vi "GetTaskStatus.vi"(8 "error in (no error)":errorcluster, 10 "task":i32, 11 "controller in":refnum<k24>) -> (0 "error out":errorcluster, 2 "task status":T1, 3 "controller out":refnum<k24>)   [LabVIEW 2010]
uses:
  c:/aerotech/controller/5.xx.xxx/A3200/pc/labview/2010/bin/Aerotech.A3200.dll
  bin/Aerotech.A3200.dll
  TaskStatus.ctl
  c:/aerotech/controller/5.xx.xxx/A3200/pc/labview/2010/bin/Aerotech.A3200.LabVIEW.dll
  bin/Aerotech.A3200.LabVIEW.dll
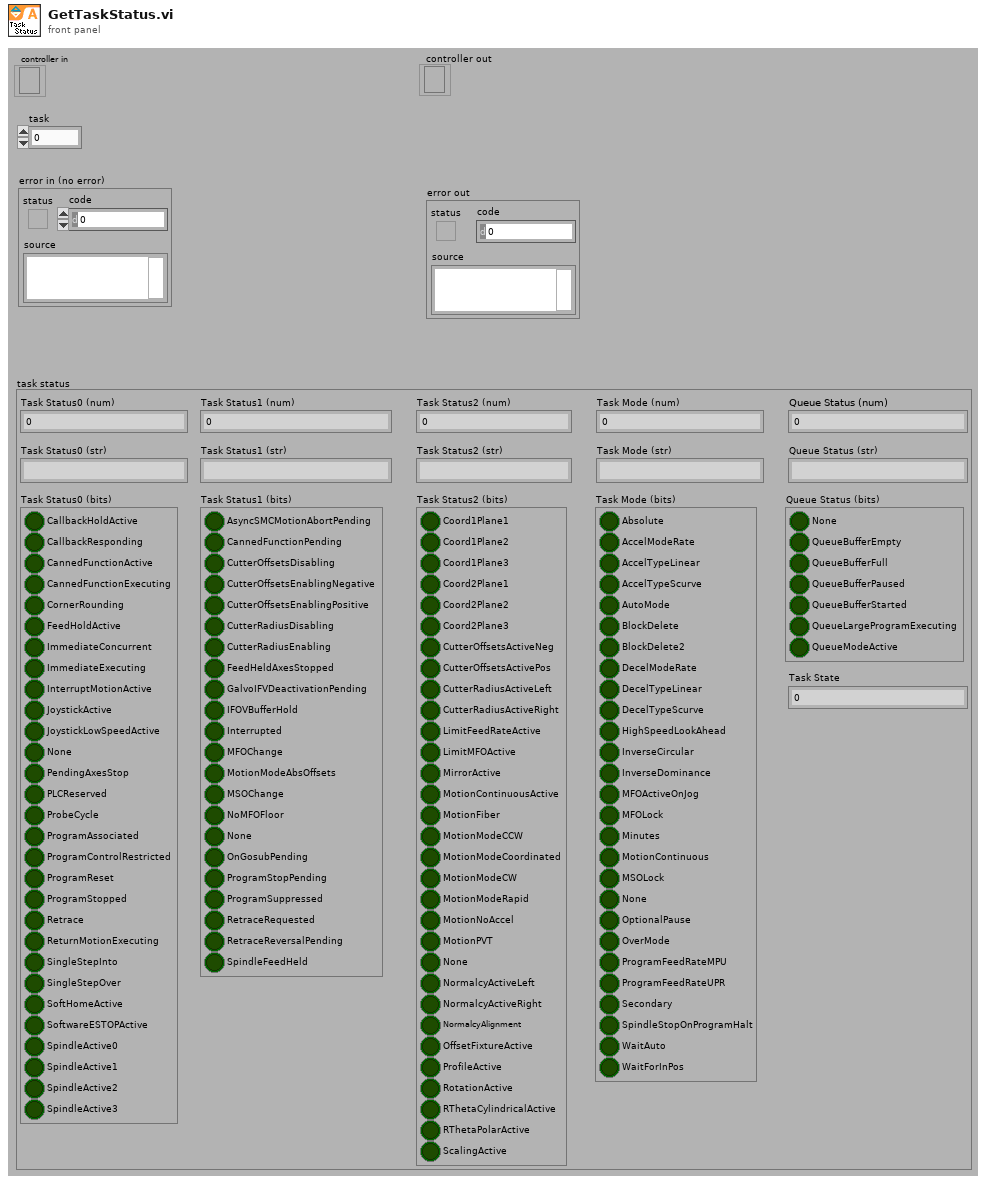
[diagram p1: front panel]
types:
  T1 = typedef "TaskStatus.ctl" = cluster{"Task Status0 (num)":i32, "Task Status0 (bits)":cluster{"CallbackHoldActive":bool, "CallbackResponding":bool, "CannedFunctionActive":bool, "CannedFunctionExecuting":bool, "CornerRounding":bool, "FeedHoldActive":bool, "ImmediateConcurrent":bool, "ImmediateExecuting":bool, "InterruptMotionActive":bool, "JoystickActive":bool, "JoystickLowSpeedActive":bool, "None":bool, "PendingAxesStop":bool, "PLCReserved":bool, "ProbeCycle":bool, "ProgramAssociated":bool, "ProgramControlRestricted":bool, "ProgramReset":bool, "ProgramStopped":bool, "Retrace":bool, "ReturnMotionExecuting":bool, "SingleStepInto":bool, "SingleStepOver":bool, "SoftHomeActive":bool, "SoftwareESTOPActive":bool, "SpindleActive0":bool, "SpindleActive1":bool, "SpindleActive2":bool, "SpindleActive3":bool}, "Task Status0 (str)":string, "Task Status1 (num)":i32, "Task Status1 (bits)":cluster{"AsyncSMCMotionAbortPending":bool, "CannedFunctionPending":bool, "CutterOffsetsDisabling":bool, "CutterOffsetsEnablingNegative":bool, "CutterOffsetsEnablingPositive":bool, "CutterRadiusDisabling":bool, "CutterRadiusEnabling":bool, "FeedHeldAxesStopped":bool, "GalvoIFVDeactivationPending":bool, "IFOVBufferHold":bool, "Interrupted":bool, "MFOChange":bool, "MotionModeAbsOffsets":bool, "MSOChange":bool, "NoMFOFloor":bool, "None":bool, "OnGosubPending":bool, "ProgramStopPending":bool, "ProgramSuppressed":bool, "RetraceRequested":bool, "RetraceReversalPending":bool, "SpindleFeedHeld":bool}, "Task Status1 (str)":string, "Task Status2 (num)":i32, "Task Status2 (bits)":cluster{"Coord1Plane1":bool, "Coord1Plane2":bool, "Coord1Plane3":bool, "Coord2Plane1":bool, "Coord2Plane2":bool, "Coord2Plane3":bool, "CutterOffsetsActiveNeg":bool, "CutterOffsetsActivePos":bool, "CutterRadiusActiveLeft":bool, "CutterRadiusActiveRight":bool, "LimitFeedRateActive":bool, "LimitMFOActive":bool, "MirrorActive":bool, "MotionContinuousActive":bool, "MotionFiber":bool, "MotionModeCCW":bool, "MotionModeCoordinated":bool, "MotionModeCW":bool, "MotionModeRapid":bool, "MotionNoAccel":bool, "MotionPVT":bool, "None":bool, "NormalcyActiveLeft":bool, "NormalcyActiveRight":bool, "NormalcyAlignment":bool, "OffsetFixtureActive":bool, "ProfileActive":bool, "RotationActive":bool, "RThetaCylindricalActive":bool, "RThetaPolarActive":bool, "ScalingActive":bool}, "Task Status2 (str)":string, "Task Mode (num)":i32, "Task Mode (bits)":cluster{"Absolute":bool, "AccelModeRate":bool, "AccelTypeLinear":bool, "AccelTypeScurve":bool, "AutoMode":bool, "BlockDelete":bool, "BlockDelete2":bool, "DecelModeRate":bool, "DecelTypeLinear":bool, "DecelTypeScurve":bool, "HighSpeedLookAhead":bool, "InverseCircular":bool, "InverseDominance":bool, "MFOActiveOnJog":bool, "MFOLock":bool, "Minutes":bool, "MotionContinuous":bool, "MSOLock":bool, "None":bool, "OptionalPause":bool, "OverMode":bool, "ProgramFeedRateMPU":bool, "ProgramFeedRateUPR":bool, "Secondary":bool, "SpindleStopOnProgramHalt":bool, "WaitAuto":bool, "WaitForInPos":bool}, "Task Mode (str)":string, "Queue Status (num)":i32, "Queue Status (bits)":cluster{"None":bool, "QueueBufferEmpty":bool, "QueueBufferFull":bool, "QueueBufferPaused":bool, "QueueBufferStarted":bool, "QueueLargeProgramExecuting":bool, "QueueModeActive":bool}, "Queue Status (str)":string, "Task State":i32}
  T2 = cluster{"taskStatus0Bits[0]":bool, "taskStatus0Bits[1]":bool, "taskStatus0Bits[2]":bool, "taskStatus0Bits[3]":bool, "taskStatus0Bits[4]":bool, "taskStatus0Bits[5]":bool, "taskStatus0Bits[6]":bool, "taskStatus0Bits[7]":bool, "taskStatus0Bits[8]":bool, "taskStatus0Bits[9]":bool, "taskStatus0Bits[10]":bool, "taskStatus0Bits[11]":bool, "taskStatus0Bits[12]":bool, "taskStatus0Bits[13]":bool, "taskStatus0Bits[14]":bool, "taskStatus0Bits[15]":bool, "taskStatus0Bits[16]":bool, "taskStatus0Bits[17]":bool, "taskStatus0Bits[18]":bool, "taskStatus0Bits[19]":bool, "taskStatus0Bits[20]":bool, "taskStatus0Bits[21]":bool, "taskStatus0Bits[22]":bool, "taskStatus0Bits[23]":bool, "taskStatus0Bits[24]":bool, "taskStatus0Bits[25]":bool, "taskStatus0Bits[26]":bool, "taskStatus0Bits[27]":bool, "taskStatus0Bits[28]":bool}
  T3 = cluster{"taskStatus1Bits[0]":bool, "taskStatus1Bits[1]":bool, "taskStatus1Bits[2]":bool, "taskStatus1Bits[3]":bool, "taskStatus1Bits[4]":bool, "taskStatus1Bits[5]":bool, "taskStatus1Bits[6]":bool, "taskStatus1Bits[7]":bool, "taskStatus1Bits[8]":bool, "taskStatus1Bits[9]":bool, "taskStatus1Bits[10]":bool, "taskStatus1Bits[11]":bool, "taskStatus1Bits[12]":bool, "taskStatus1Bits[13]":bool, "taskStatus1Bits[14]":bool, "taskStatus1Bits[15]":bool, "taskStatus1Bits[16]":bool, "taskStatus1Bits[17]":bool, "taskStatus1Bits[18]":bool, "taskStatus1Bits[19]":bool, "taskStatus1Bits[20]":bool, "taskStatus1Bits[21]":bool}
  T4 = cluster{"taskStatus2Bits[0]":bool, "taskStatus2Bits[1]":bool, "taskStatus2Bits[2]":bool, "taskStatus2Bits[3]":bool, "taskStatus2Bits[4]":bool, "taskStatus2Bits[5]":bool, "taskStatus2Bits[6]":bool, "taskStatus2Bits[7]":bool, "taskStatus2Bits[8]":bool, "taskStatus2Bits[9]":bool, "taskStatus2Bits[10]":bool, "taskStatus2Bits[11]":bool, "taskStatus2Bits[12]":bool, "taskStatus2Bits[13]":bool, "taskStatus2Bits[14]":bool, "taskStatus2Bits[15]":bool, "taskStatus2Bits[16]":bool, "taskStatus2Bits[17]":bool, "taskStatus2Bits[18]":bool, "taskStatus2Bits[19]":bool, "taskStatus2Bits[20]":bool, "taskStatus2Bits[21]":bool, "taskStatus2Bits[22]":bool, "taskStatus2Bits[23]":bool, "taskStatus2Bits[24]":bool, "taskStatus2Bits[25]":bool, "taskStatus2Bits[26]":bool, "taskStatus2Bits[27]":bool, "taskStatus2Bits[28]":bool, "taskStatus2Bits[29]":bool, "taskStatus2Bits[30]":bool}
  T5 = cluster{"taskModeBits[0]":bool, "taskModeBits[1]":bool, "taskModeBits[2]":bool, "taskModeBits[3]":bool, "taskModeBits[4]":bool, "taskModeBits[5]":bool, "taskModeBits[6]":bool, "taskModeBits[7]":bool, "taskModeBits[8]":bool, "taskModeBits[9]":bool, "taskModeBits[10]":bool, "taskModeBits[11]":bool, "taskModeBits[12]":bool, "taskModeBits[13]":bool, "taskModeBits[14]":bool, "taskModeBits[15]":bool, "taskModeBits[16]":bool, "taskModeBits[17]":bool, "taskModeBits[18]":bool, "taskModeBits[19]":bool, "taskModeBits[20]":bool, "taskModeBits[21]":bool, "taskModeBits[22]":bool, "taskModeBits[23]":bool, "taskModeBits[24]":bool, "taskModeBits[25]":bool, "taskModeBits[26]":bool}
  T6 = cluster{"queueStatusBits[0]":bool, "queueStatusBits[1]":bool, "queueStatusBits[2]":bool, "queueStatusBits[3]":bool, "queueStatusBits[4]":bool, "queueStatusBits[5]":bool, "queueStatusBits[6]":bool}
  T7 = cluster{"taskStatus0MaskValue":i32, "taskStatus0Bits":cluster{"taskStatus0Bits[0]":bool, "taskStatus0Bits[1]":bool, "taskStatus0Bits[2]":bool, "taskStatus0Bits[3]":bool, "taskStatus0Bits[4]":bool, "taskStatus0Bits[5]":bool, "taskStatus0Bits[6]":bool, "taskStatus0Bits[7]":bool, "taskStatus0Bits[8]":bool, "taskStatus0Bits[9]":bool, "taskStatus0Bits[10]":bool, "taskStatus0Bits[11]":bool, "taskStatus0Bits[12]":bool, "taskStatus0Bits[13]":bool, "taskStatus0Bits[14]":bool, "taskStatus0Bits[15]":bool, "taskStatus0Bits[16]":bool, "taskStatus0Bits[17]":bool, "taskStatus0Bits[18]":bool, "taskStatus0Bits[19]":bool, "taskStatus0Bits[20]":bool, "taskStatus0Bits[21]":bool, "taskStatus0Bits[22]":bool, "taskStatus0Bits[23]":bool, "taskStatus0Bits[24]":bool, "taskStatus0Bits[25]":bool, "taskStatus0Bits[26]":bool, "taskStatus0Bits[27]":bool, "taskStatus0Bits[28]":bool}, "taskStatus0String":string, "taskStatus1MaskValue":i32, "taskStatus1Bits":cluster{"taskStatus1Bits[0]":bool, "taskStatus1Bits[1]":bool, "taskStatus1Bits[2]":bool, "taskStatus1Bits[3]":bool, "taskStatus1Bits[4]":bool, "taskStatus1Bits[5]":bool, "taskStatus1Bits[6]":bool, "taskStatus1Bits[7]":bool, "taskStatus1Bits[8]":bool, "taskStatus1Bits[9]":bool, "taskStatus1Bits[10]":bool, "taskStatus1Bits[11]":bool, "taskStatus1Bits[12]":bool, "taskStatus1Bits[13]":bool, "taskStatus1Bits[14]":bool, "taskStatus1Bits[15]":bool, "taskStatus1Bits[16]":bool, "taskStatus1Bits[17]":bool, "taskStatus1Bits[18]":bool, "taskStatus1Bits[19]":bool, "taskStatus1Bits[20]":bool, "taskStatus1Bits[21]":bool}, "taskStatus1String":string, "taskStatus2MaskValue":i32, "taskStatus2Bits":cluster{"taskStatus2Bits[0]":bool, "taskStatus2Bits[1]":bool, "taskStatus2Bits[2]":bool, "taskStatus2Bits[3]":bool, "taskStatus2Bits[4]":bool, "taskStatus2Bits[5]":bool, "taskStatus2Bits[6]":bool, "taskStatus2Bits[7]":bool, "taskStatus2Bits[8]":bool, "taskStatus2Bits[9]":bool, "taskStatus2Bits[10]":bool, "taskStatus2Bits[11]":bool, "taskStatus2Bits[12]":bool, "taskStatus2Bits[13]":bool, "taskStatus2Bits[14]":bool, "taskStatus2Bits[15]":bool, "taskStatus2Bits[16]":bool, "taskStatus2Bits[17]":bool, "taskStatus2Bits[18]":bool, "taskStatus2Bits[19]":bool, "taskStatus2Bits[20]":bool, "taskStatus2Bits[21]":bool, "taskStatus2Bits[22]":bool, "taskStatus2Bits[23]":bool, "taskStatus2Bits[24]":bool, "taskStatus2Bits[25]":bool, "taskStatus2Bits[26]":bool, "taskStatus2Bits[27]":bool, "taskStatus2Bits[28]":bool, "taskStatus2Bits[29]":bool, "taskStatus2Bits[30]":bool}, "taskStatus2String":string, "taskModeMaskValue":i32, "taskModeBits":cluster{"taskModeBits[0]":bool, "taskModeBits[1]":bool, "taskModeBits[2]":bool, "taskModeBits[3]":bool, "taskModeBits[4]":bool, "taskModeBits[5]":bool, "taskModeBits[6]":bool, "taskModeBits[7]":bool, "taskModeBits[8]":bool, "taskModeBits[9]":bool, "taskModeBits[10]":bool, "taskModeBits[11]":bool, "taskModeBits[12]":bool, "taskModeBits[13]":bool, "taskModeBits[14]":bool, "taskModeBits[15]":bool, "taskModeBits[16]":bool, "taskModeBits[17]":bool, "taskModeBits[18]":bool, "taskModeBits[19]":bool, "taskModeBits[20]":bool, "taskModeBits[21]":bool, "taskModeBits[22]":bool, "taskModeBits[23]":bool, "taskModeBits[24]":bool, "taskModeBits[25]":bool, "taskModeBits[26]":bool}, "taskModeString":string, "queueStatusMaskValue":i32, "queueStatusBits":cluster{"queueStatusBits[0]":bool, "queueStatusBits[1]":bool, "queueStatusBits[2]":bool, "queueStatusBits[3]":bool, "queueStatusBits[4]":bool, "queueStatusBits[5]":bool, "queueStatusBits[6]":bool}, "queueStatusString":string, "taskState":i32}
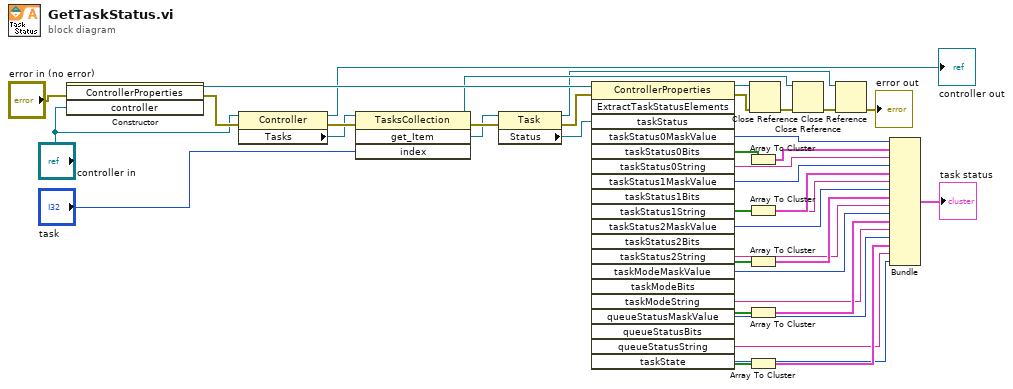
[diagram p0: block diagram]
diagram:
  n1 = constructor class="ControllerProperties"(error in="error in (no error)", "controller"="controller in") -> (reference out=w40:refnum<k24>, error out=w39:errorcluster)  [unwired: 2 in, 2 out]
  n2 = property class="Controller"(reference="controller in", error in=w39) -> (reference out=→"controller out":refnum<k24>, error out=w37:errorcluster, "Tasks"=w9:refnum<k24>)
  n3 = invoke class="TasksCollection" method="get_Item"(reference=w9, error in=w37, "index"="task") -> (reference out=w5:refnum<k24>, error out=w35:errorcluster, "get_Item"=w34:refnum<k24>)  [unwired: 1 in, 1 out]
  n4 = property class="Task"(reference=w34, error in=w35) -> (reference out=w4:refnum<k24>, error out=w32:errorcluster, "Status"=w33:refnum<k24>)
  n5 = invoke class="ControllerProperties" method="ExtractTaskStatusElements"(reference=w40, error in=w32, "taskStatus"=w33) -> (reference out=w7:refnum<k24>, error out=w6:errorcluster, "taskStatus0MaskValue"=w31:i32, "taskStatus0Bits"=w30:bool[], "taskStatus0String"=w24:string, "taskStatus1MaskValue"=w23:i32, "taskStatus1Bits"=w29:bool[], "taskStatus1String"=w21:string, "taskStatus2MaskValue"=w20:i32, "taskStatus2Bits"=w28:bool[], "taskStatus2String"=w18:string, "taskModeMaskValue"=w17:i32, "taskModeBits"=w27:bool[], "taskModeString"=w15:string, "queueStatusMaskValue"=w14:i32, "queueStatusBits"=w26:bool[], "queueStatusString"=w12:string, "taskState"=w11:i32)  [unwired: 17 in, 2 out]
  n6 = Array To Cluster(array=w30) -> (cluster=w25:T2)
  n7 = Array To Cluster(array=w29) -> (cluster=w22:T3)
  n8 = Array To Cluster(array=w28) -> (cluster=w19:T4)
  n9 = Array To Cluster(array=w27) -> (cluster=w16:T5)
  n10 = Array To Cluster(array=w26) -> (cluster=w13:T6)
  n11 = Close Reference(reference=w7, error in (no error)=w6) -> (error out=w3:errorcluster)
  n12 = Close Reference(reference=w5, error in (no error)=w3) -> (error out=w2:errorcluster)
  n13 = Close Reference(reference=w4, error in (no error)=w2) -> (error out=→"error out":errorcluster)
  n14 = Bundle("taskStatus0MaskValue"=w31, "taskStatus0Bits"=w25, "taskStatus0String"=w24, "taskStatus1MaskValue"=w23, "taskStatus1Bits"=w22, "taskStatus1String"=w21, "taskStatus2MaskValue"=w20, "taskStatus2Bits"=w19, "taskStatus2String"=w18, "taskModeMaskValue"=w17, "taskModeBits"=w16, "taskModeString"=w15, "queueStatusMaskValue"=w14, "queueStatusBits"=w13, "queueStatusString"=w12, "taskState"=w11) -> (→"task status":T7)  [unwired: 1 in]
